vi "Measurement UI.vi"() -> ()   [LabVIEW 2021, in "Single Tone Measurements_Class D Amplifier.lvlib"]
uses:
  Single Tone Measurements_Class D Amplifier.lvlib
  shared/controls/units - snr.ctl
  shared/controls/units - ratio.ctl
  shared/controls/audio controls.lvlib
panel:
  in  "Graphs":enum32{"Frequency Domain", "Time Domain"}(tab)
  out "frequency domain":T1(graph)
  out "time domain":waveform(dbl)(graph)
  out "meas table":string[][](table)
  out "amplitude (Vrms)":dbl
  out "output power (W)":dbl
  in  "Configuration tab":enum32{"Protocol", "Measurement", "Units"}(tab)
  in  "master clock channel list":string caption="Master Clock Channel"
  in  "digital channel list":string caption="Digital Audio Channel"
  in  "logic level":enum32{"3.3 V", "1.8 V", "1.2 V"}(ring) caption="Logic level"
  in  "master clock rate":dbl=12288000.0 caption="Master clock rate" format="%#_6pHz"
  out "Bit clock rate":dbl=3072000.0 format="%#_6pHz"
  in  "number of channels":u8=2 caption="Number of channels"
  in  "TDM":bool
  in  "RJ":bool
  in  "LJ":bool
  in  "I2S":bool
  in  "bit clock edge sync":enum32{"Rising", "Falling"}(ring)=enum."Falling" caption="Bit clock edge sync"
  in  "frame clock rate":dbl=48000.0 caption="Frame clock rate" format="%#_6pHz"
  in  "data justification":enum32{"Left Justified", "Right Justified"}(ring) caption="Data justification"
  in  "endianness":enum32{"MSB First", "LSB First"}(ring) caption="Endianness"
  in  "bit depth":u8=24 caption="Bit depth"
  in  "channel length":u16=32 caption="Channel length"
  in  "frame sync edge for channel 0":enum32{"Rising", "Falling"}(ring)=enum."Falling" caption="Frame sync edge for Channel 0"
  in  "min settling cycles":u32 caption="Minimum settling cycles"
  in  "min settling time (s)":dbl=0.1 caption="Minimum settling time" format="%#_6ps"
  in  "min measurement cycles":u32 caption="Minimum measurement cycles"
  in  "min measurement time (s)":dbl=0.1 caption="Minimum measurement time" format="%#_6ps"
  in  "output power (W)":dbl=1.0 caption="Output power" format="%#_6p W"
  in  "output mode":enum16{"Level", "Power"}(ring) caption="Output mode"
  in  "Acquisition channel":tag
  in  "acq sampling rate":dbl=51200.0 caption="Sample rate" format="%#.6pHz"
  in  "lowpass filter":T2(ring) caption="Lowpass filter"
  in  "highpass filter":enum32{"DC", "AC"}(ring) caption="Highpass filter"
  in  "band start":dbl=20.0 caption="Band start" format="%#_6pHz"
  in  "band stop":dbl=20000.0 caption="Band stop" format="%#_6pHz"
  in  "weighting filter":T3(ring)=enum."A-weighting" caption="Weighting filter"
  in  "load impedance":dbl=4.0 caption="Load impedance" format="%#_6p Ohms"
  in  "output range (pk-pk)":dbl=15.0 caption="Output range" format="%.3p Vpk-pk"
  in  "signal frequency":dbl=1000.0 caption="Frequency" format="%#_6pHz"
  in  "output level (dB)":dbl=-1.0 caption="Output level" format="%#_6p dBFS"
  in  "testDBL":dbl
  in  "gain units":T4 caption="Gain"
  in  "THD units":T4 caption="THD"
  in  "THD+N units":T4 caption="THD+N"
  in  "SNR units":T5 caption="SNR"
  in  "channel 0 offset":u32=1
  out "fft - data":dbl[](array[numeric])
  out "fft - df":dbl
  out "fft - f0":dbl
  out "wfm - data":dbl[](array[numeric])
  out "wfm - dt":dbl
  out "wfm - t0":dbl
  out "SFDR (dBc)":dbl
  out "gain":dbl
  out "dynamic range (dB)":dbl
  out "THD":dbl
  out "THD+N":dbl
  out "SNR":dbl
  out "amplitude (dBFS)":dbl
  out "frequency (Hz)":dbl
  out "channel name":string
  in  "acq channel":string="PXI1Slot4/ai0"
  in  "signal phase":dbl caption="phase"
  # "hidden controls - used to sync with MeasLink"
  # "hidden indicators"
  # "Protocols"
  # "Audio Protocol"
  # "Clock Settings"
  # "Signal Level"
  # "Harware Resource"
  # "Filters"
  # "Output"
  # "Acquisition"
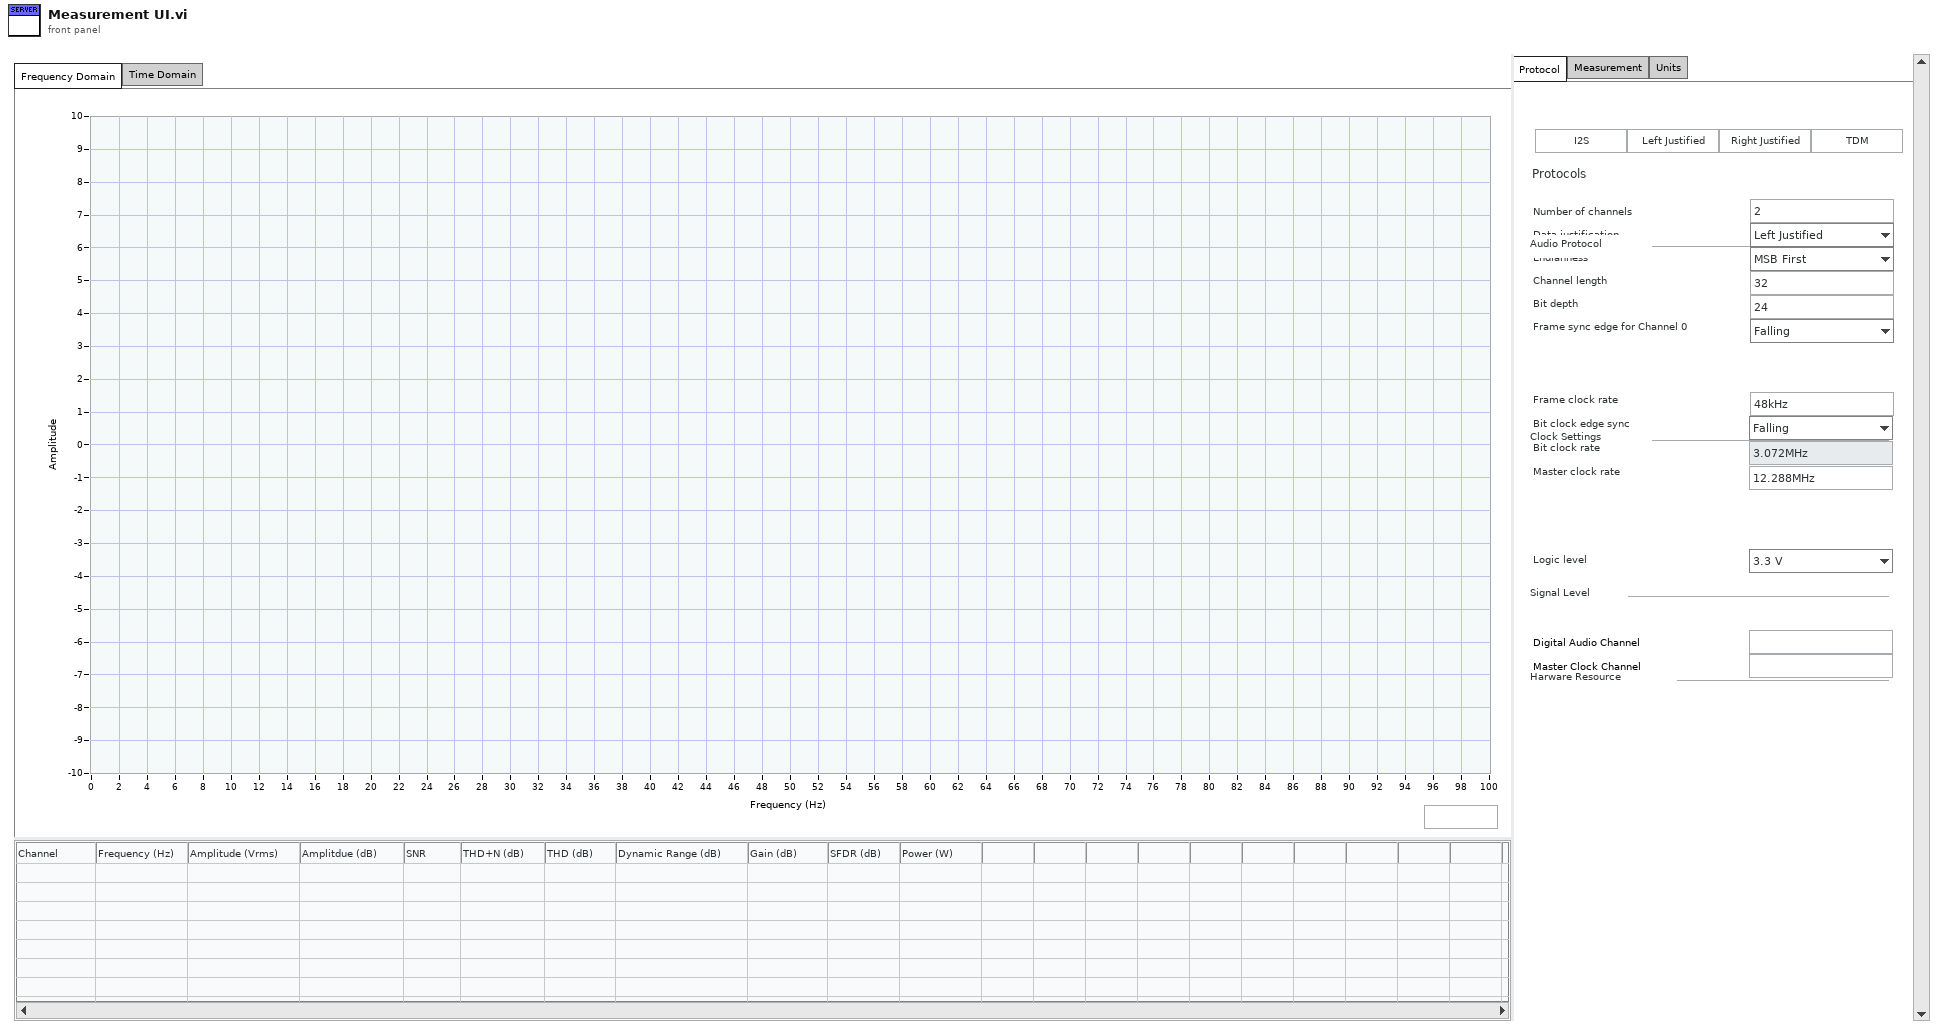
[diagram p1: front panel]
types:
  T1 = cluster{"fft - f0":dbl, "fft - df":dbl, "fft - data":dbl[]}
  T2 = enum32{"No filter", "AES17 20kHz", "AES17 40kHz"}
  T3 = enum32{"Linear", "A-weighting", "B-weighting", "C-weighting"}
  T4 = typedef "audio controls.lvlib/units - ratio.ctl" = enum16{"dB", "%", "x/y"}
  T5 = typedef "audio controls.lvlib/units - snr.ctl" = enum16{"dB", "x/y"}
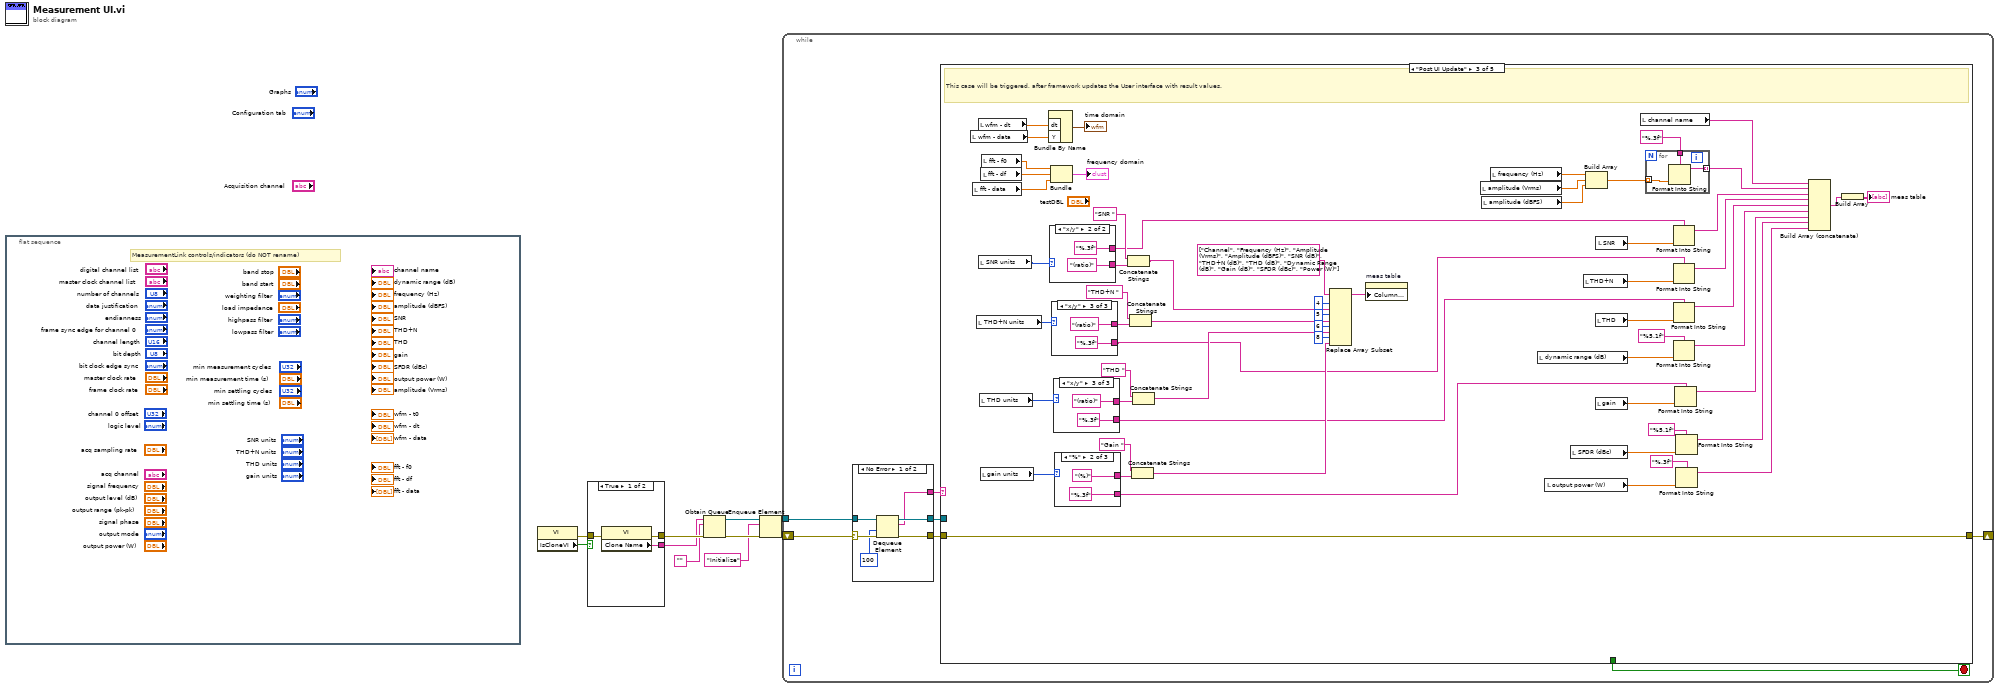
[diagram p0: block diagram]
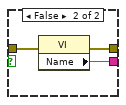
[diagram p2: hidden frame]
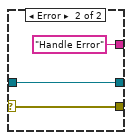
[diagram p3: hidden frame]
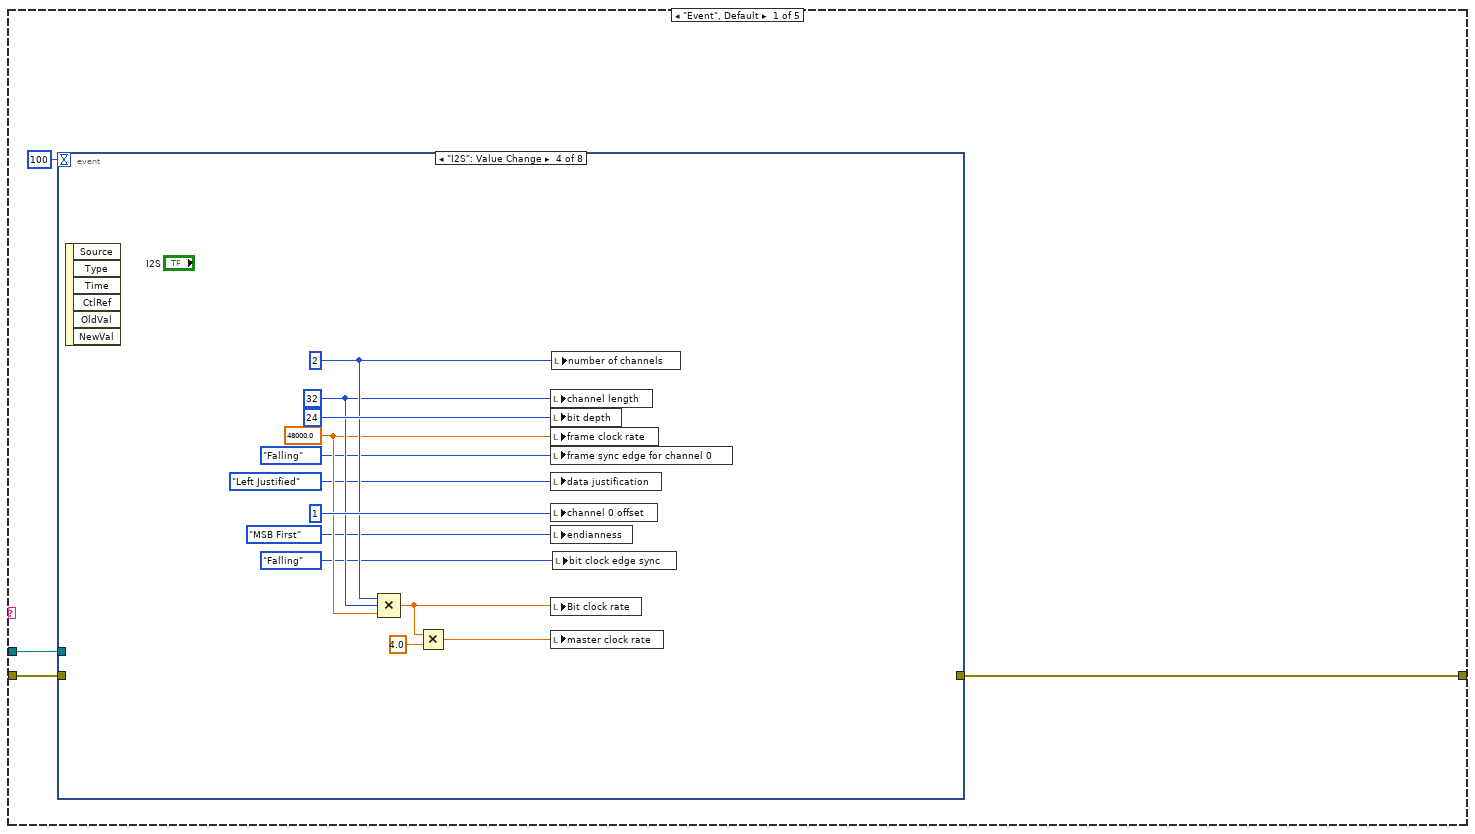
[diagram p4: hidden frame]
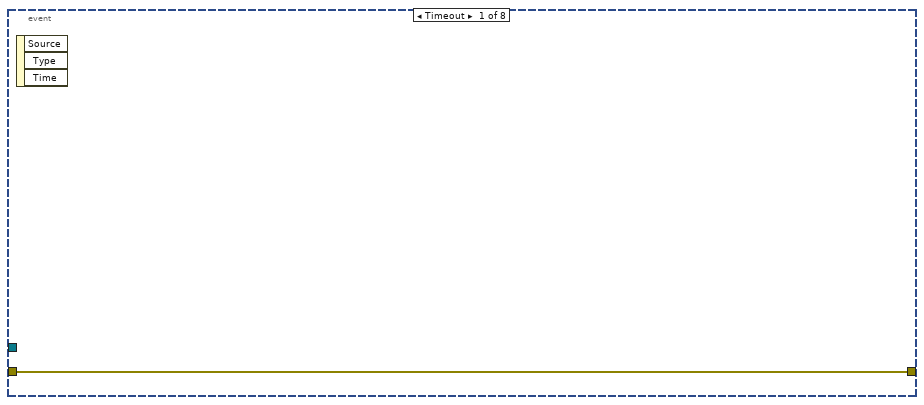
[diagram p5: hidden frame]
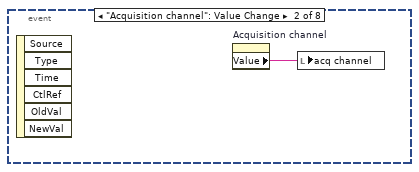
[diagram p6: hidden frame]
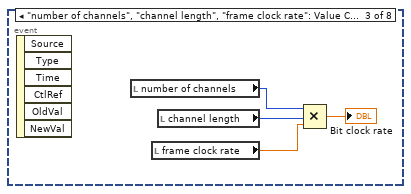
[diagram p7: hidden frame]
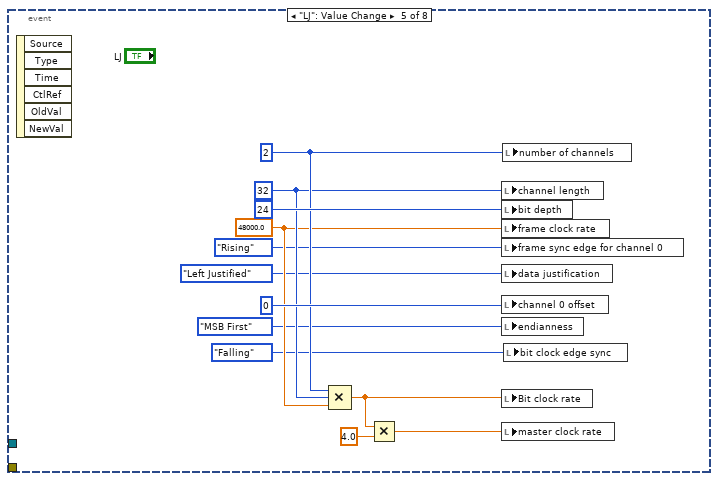
[diagram p8: hidden frame]
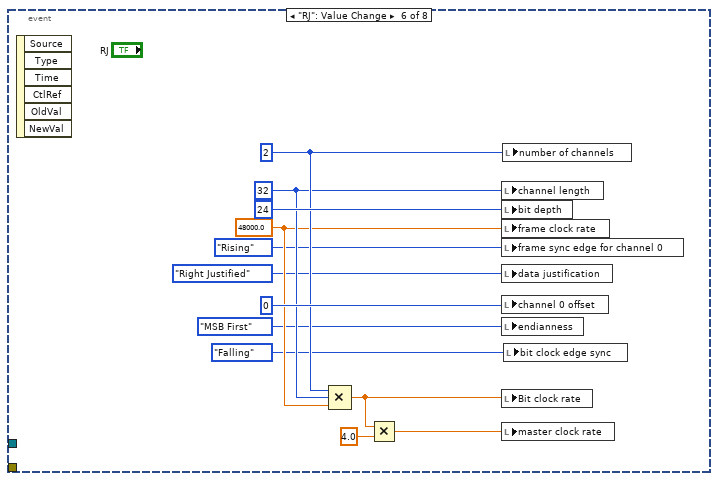
[diagram p9: hidden frame]
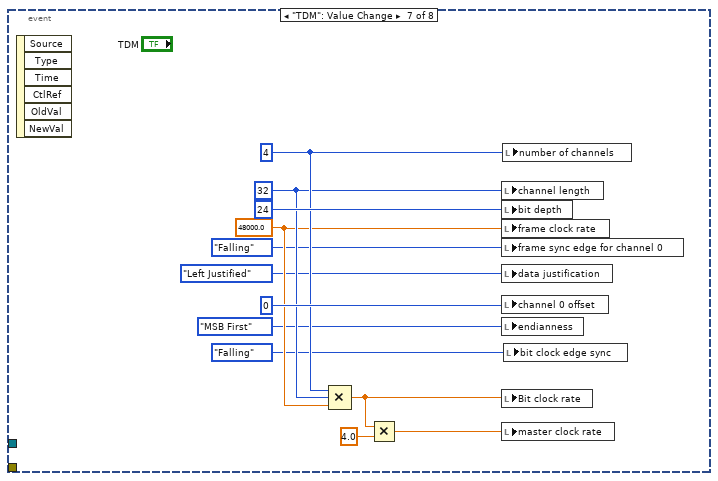
[diagram p10: hidden frame]
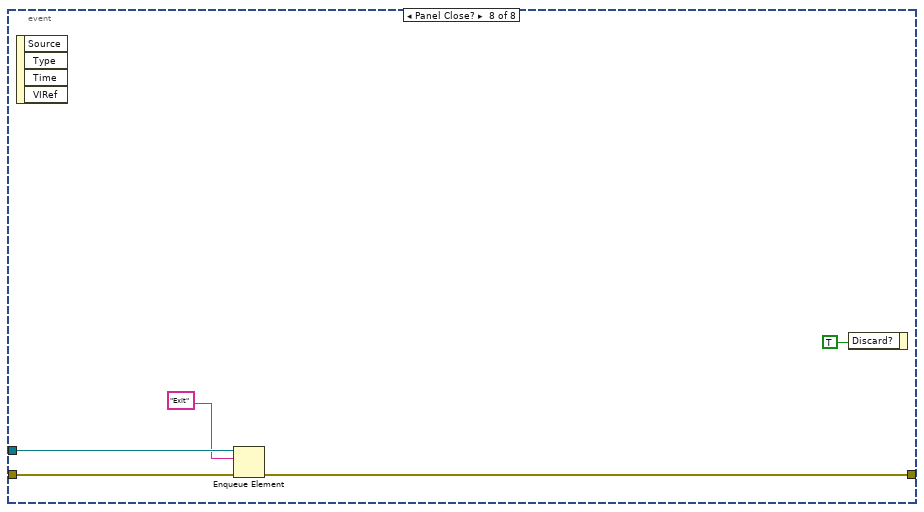
[diagram p11: hidden frame]
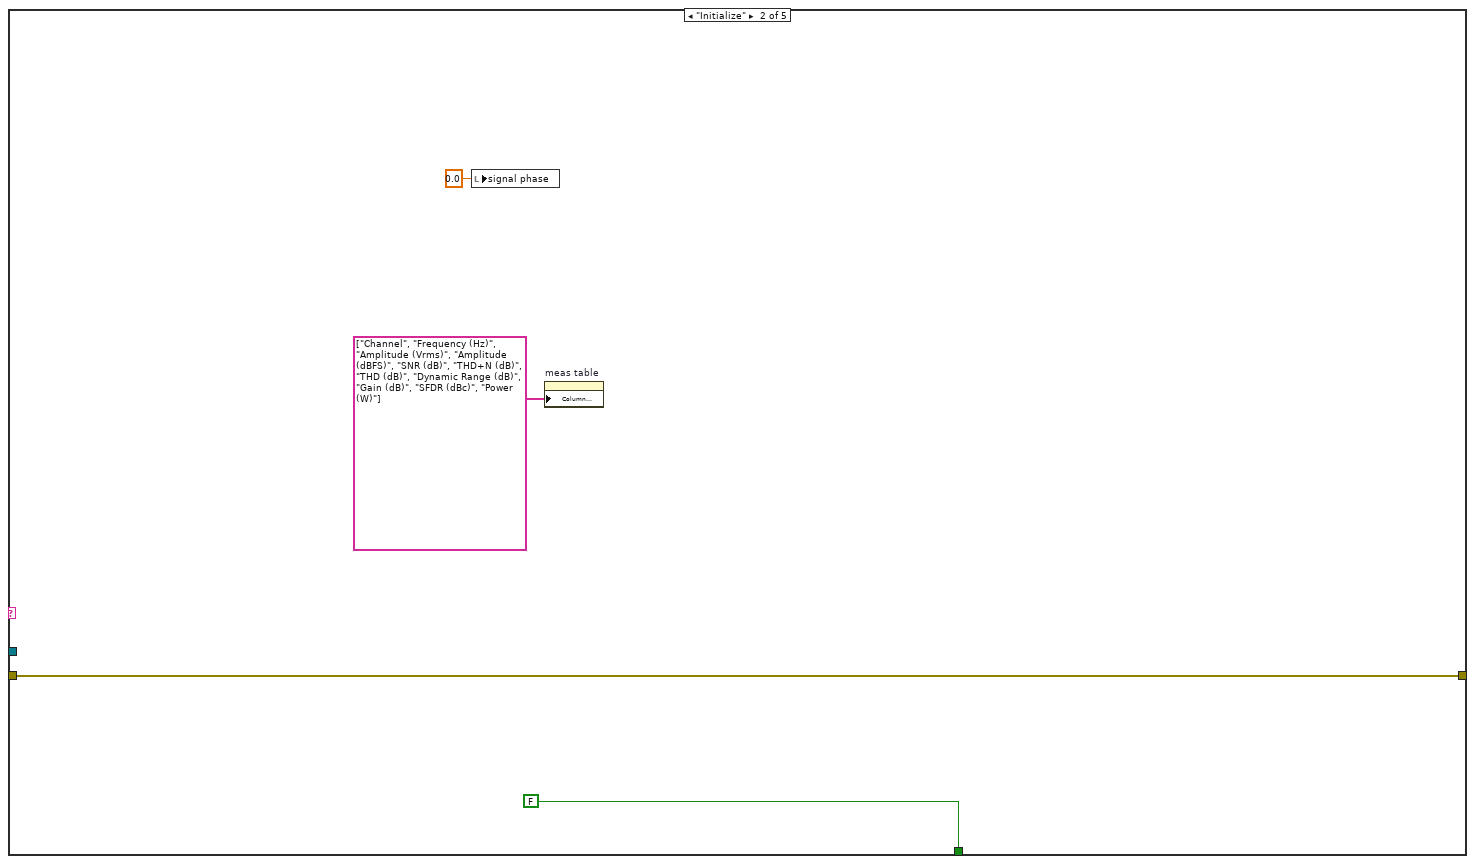
[diagram p12: hidden frame]
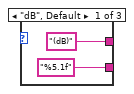
[diagram p13: hidden frame]
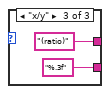
[diagram p14: hidden frame]
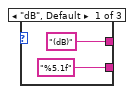
[diagram p15: hidden frame]
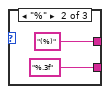
[diagram p16: hidden frame]
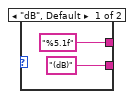
[diagram p17: hidden frame]
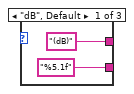
[diagram p18: hidden frame]
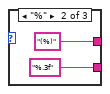
[diagram p19: hidden frame]
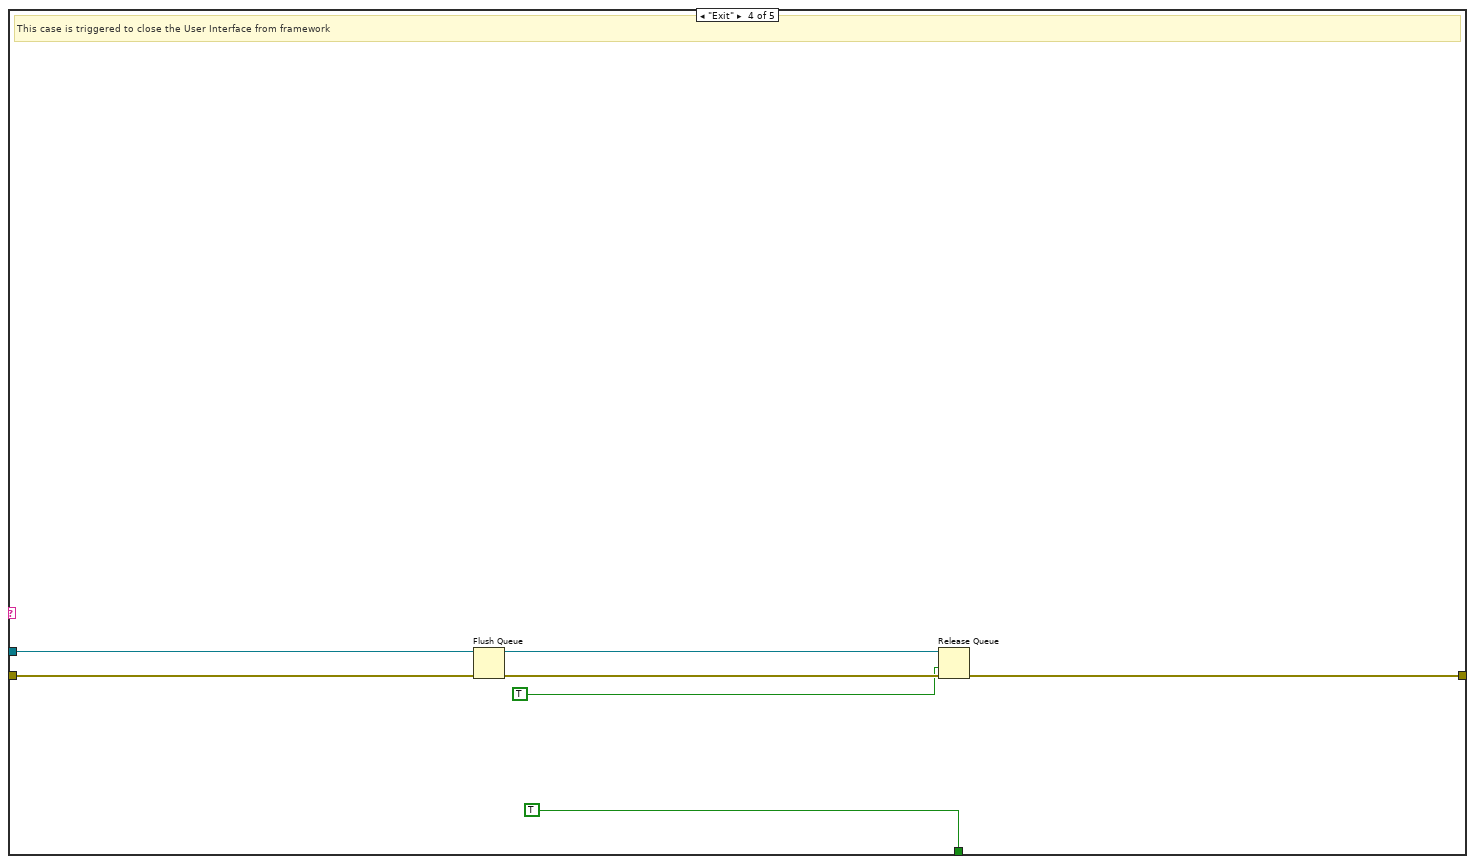
[diagram p20: hidden frame]
diagram:
  n1 = flat-sequence {
    frame #0 {
      # "MeasurementLink controls/indicators (do NOT rename)"
    }
  }
  n2 = property class="VI"() -> (error out=w1:errorcluster, "IsCloneVI"=w2:bool)  [unwired: 2 in, 1 out]
  n3 = case shown="True" w2 {
    tunnel: [w13 w16] -> w10
    tunnel: [w12 w15] -> w9
    tunnel: w1 -> [w11 w14]
    frame True {
      n4 = property class="VI"(error in=w11) -> (error out=w13:errorcluster, "Clone Name"=w12:string)  [unwired: 1 in, 1 out]
    }
    frame False {
      n5 = property class="VI"(error in=w14) -> (error out=w16:errorcluster, "Name"=w15:string)  [unwired: 1 in, 1 out]
    }
  }
  n6 = Obtain Queue(name (unnamed)=w9, element data type="", error in (no error)=w10) -> (queue out=w6:refnum<queue>, error out=w8:errorcluster)  [unwired: 2 in, 1 out]
  n7 = Enqueue Element(queue=w6, element="Initialize", error in (no error)=w8) -> (queue out=w5:refnum<queue>, error out=w7:errorcluster)  [unwired: 1 in, 1 out]
  n8 = while {
    shift-right: [w18] -> _
    shift-left: w7 -> [w23]
    tunnel: w5 -> [w21]
    stop <- w17 stop-if-true
    n9 = case shown="No Error" w23 {
      selector: w23 -> [w29 w32]
      tunnel: [w28 w32] -> w22
      tunnel: w21 -> [w27 w31]
      tunnel: [w26 w31] -> w20
      tunnel: [w25 "Handle Error"] -> w19
      frame No Error {
        n10 = Dequeue Element(queue=w27, timeout in ms (-1)=100, error in (no error)=w29) -> (queue out=w26:refnum<queue>, element=w25:string, error out=w28:errorcluster)  [unwired: 1 out]
      }
      frame Error {
      }
    }
    n11 = case shown="\"Post UI Update\"" w19 {
      tunnel: w22 -> [w35 w99 w159 w191 w192]
      tunnel: w20 -> [w33 _ _ w189 _]
      tunnel: [w36 w99 w159 w186 w192] -> w18
      tunnel: [_ FALSE _ TRUE _] -> w17
      frame "Event", Default {
        n12 = event shown="[3] \"I2S\": Value Change" {
          selector: _ -> [_ _ _ _ _ _ _ _]
          dyn-events: _ -> [_ _ _ _ _ _ _ _]
          timeout: 100 -> [_ _ _ _ _ _ _ _]
          tunnel: [w37 _ _ _ _ _ _ w93] -> w36
          tunnel: w35 -> [w37 _ _ _ _ _ _ w94]
          tunnel: w33 -> [_ _ _ _ _ _ _ w92]
          event Timeout {
            n13 = event-data() -> ()  [unwired: 1 in, 3 out]
          }
          event "Acquisition channel": Value Change {
            n14 = event-data() -> ()  [unwired: 1 in, 6 out]
            n15 = property on="Acquisition channel" class="DAQmxName"() -> ("Value"=w38:string)  [unwired: 2 in, 2 out]
            n16 = local write "acq channel"(w38) -> ()
          }
          event "number of channels", "channel length", "frame clock rate": Value Change {
            n17 = event-data() -> ()  [unwired: 1 in, 6 out]
            n18 = local read "number of channels"() -> (w42:u8)
            n19 = local read "frame clock rate"() -> (w40:dbl)
            n20 = local read "channel length"() -> (w41:u16)
            n21 = Compound Arithmetic op=MULTIPLY(w42, w41, w40) -> (→"Bit clock rate":dbl)
          }
          event "I2S": Value Change {
            w50 = 48000.0 ("Frame Clock Rate")
            w51 = u32 32 ("Channel Length")
            w52 = u32 2 ("Number of Channels")
            n22 = event-data() -> ()  [unwired: 1 in, 6 out]
            n23 = Compound Arithmetic op=MULTIPLY(w52, w51, w50) -> (w49:dbl)
            n24 = Multiply(x=w49, y=4.0) -> (x*y=w48:dbl)
            n25 = local write "channel length"(w51) -> ()
            n26 = local write "bit depth"(u32 24 ("Bit Depth")) -> ()
            n27 = local write "frame clock rate"(w50) -> ()
            n28 = local write "frame sync edge for channel 0"(enum32{"Rising", "Falling"}."Falling" ("bit clock edge sync")) -> ()
            n29 = local write "data justification"(enum32{"Left Justified", "Right Justified"}."Left Justified" ("data justification")) -> ()
            n30 = local write "channel 0 offset"(u32 1 ("Channel 0 Offset")) -> ()
            n31 = local write "endianness"(enum32{"MSB First", "LSB First"}."MSB First" ("endianness")) -> ()
            n32 = local write "Bit clock rate"(w49) -> ()
            n33 = local write "master clock rate"(w48) -> ()
            n34 = local write "number of channels"(w52) -> ()
            n35 = local write "bit clock edge sync"(enum32{"Rising", "Falling"}."Falling" ("frame sync edge for channel 0")) -> ()
          }
          event "LJ": Value Change {
            w62 = 48000.0 ("Frame Clock Rate")
            w63 = u32 32 ("Channel Length")
            w64 = u32 2 ("Number of Channels")
            n36 = event-data() -> ()  [unwired: 1 in, 6 out]
            n37 = Compound Arithmetic op=MULTIPLY(w64, w63, w62) -> (w61:dbl)
            n38 = Multiply(x=w61, y=4.0) -> (x*y=w60:dbl)
            n39 = local write "channel length"(w63) -> ()
            n40 = local write "bit depth"(u32 24 ("Bit Depth")) -> ()
            n41 = local write "frame clock rate"(w62) -> ()
            n42 = local write "frame sync edge for channel 0"(enum32{"Rising", "Falling"}."Rising" ("bit clock edge sync")) -> ()
            n43 = local write "data justification"(enum32{"Left Justified", "Right Justified"}."Left Justified" ("data justification")) -> ()
            n44 = local write "channel 0 offset"(u32 0 ("Channel 0 Offset")) -> ()
            n45 = local write "endianness"(enum32{"MSB First", "LSB First"}."MSB First" ("endianness")) -> ()
            n46 = local write "Bit clock rate"(w61) -> ()
            n47 = local write "master clock rate"(w60) -> ()
            n48 = local write "number of channels"(w64) -> ()
            n49 = local write "bit clock edge sync"(enum32{"Rising", "Falling"}."Falling" ("frame sync edge for channel 0")) -> ()
          }
          event "RJ": Value Change {
            w74 = 48000.0 ("Frame Clock Rate")
            w75 = u32 32 ("Channel Length")
            w76 = u32 2 ("Number of Channels")
            n50 = event-data() -> ()  [unwired: 1 in, 6 out]
            n51 = Compound Arithmetic op=MULTIPLY(w76, w75, w74) -> (w73:dbl)
            n52 = Multiply(x=w73, y=4.0) -> (x*y=w72:dbl)
            n53 = local write "channel length"(w75) -> ()
            n54 = local write "bit depth"(u32 24 ("Bit Depth")) -> ()
            n55 = local write "frame clock rate"(w74) -> ()
            n56 = local write "frame sync edge for channel 0"(enum32{"Rising", "Falling"}."Rising" ("bit clock edge sync")) -> ()
            n57 = local write "data justification"(enum32{"Left Justified", "Right Justified"}."Right Justified" ("data justification")) -> ()
            n58 = local write "channel 0 offset"(u32 0 ("Channel 0 Offset")) -> ()
            n59 = local write "endianness"(enum32{"MSB First", "LSB First"}."MSB First" ("endianness")) -> ()
            n60 = local write "Bit clock rate"(w73) -> ()
            n61 = local write "master clock rate"(w72) -> ()
            n62 = local write "number of channels"(w76) -> ()
            n63 = local write "bit clock edge sync"(enum32{"Rising", "Falling"}."Falling" ("frame sync edge for channel 0")) -> ()
          }
          event "TDM": Value Change {
            w86 = 48000.0 ("Frame Clock Rate")
            w87 = u32 32 ("Channel Length")
            w88 = u32 4 ("Number of Channels")
            n64 = event-data() -> ()  [unwired: 1 in, 6 out]
            n65 = Compound Arithmetic op=MULTIPLY(w88, w87, w86) -> (w85:dbl)
            n66 = Multiply(x=w85, y=4.0) -> (x*y=w84:dbl)
            n67 = local write "channel length"(w87) -> ()
            n68 = local write "bit depth"(u32 24 ("Bit Depth")) -> ()
            n69 = local write "frame clock rate"(w86) -> ()
            n70 = local write "frame sync edge for channel 0"(enum32{"Rising", "Falling"}."Falling" ("bit clock edge sync")) -> ()
            n71 = local write "data justification"(enum32{"Left Justified", "Right Justified"}."Left Justified" ("data justification")) -> ()
            n72 = local write "channel 0 offset"(u32 0 ("Channel 0 Offset")) -> ()
            n73 = local write "endianness"(enum32{"MSB First", "LSB First"}."MSB First" ("endianness")) -> ()
            n74 = local write "Bit clock rate"(w85) -> ()
            n75 = local write "master clock rate"(w84) -> ()
            n76 = local write "number of channels"(w88) -> ()
            n77 = local write "bit clock edge sync"(enum32{"Rising", "Falling"}."Falling" ("frame sync edge for channel 0")) -> ()
          }
          event Panel Close? {
            n78 = event-data() -> ()  [unwired: 1 in, 4 out]
            n79 = Enqueue Element(queue=w92, element="Exit", error in (no error)=w94) -> (error out=w93:errorcluster)  [unwired: 1 in, 2 out]
            n80 = event-data("Discard?"=TRUE) -> ()  [unwired: 1 in, 1 out]
          }
        }
      }
      frame "Initialize" {
        n81 = local write "signal phase"(0.0 ("signal phase")) -> ()
        n82 = property on="meas table" class="Tbl (strict)"("Column Headers[]"=string[] ["Channel", "Frequency (Hz)", "Amplitude (Vrms)", "Amplitude (dBFS)", "SNR (dB)", "THD+N (dB)", "THD (dB)", "Dynamic Range (dB)", "Gain (dB)", "SFDR (dBc)", "Power (W)"] ("Column Header Strings[]")) -> ()  [unwired: 2 in, 2 out]
      }
      frame "Post UI Update" {
        # "This case will be triggered, after framework updates the User interface with result values."
        n83 = local read "wfm - data"() -> (w157:dbl[])
        n84 = local read "fft - data"() -> (w153:dbl[])
        n85 = local read "THD+N units"() -> (w132:T4)
        n86 = local read "wfm - dt"() -> (w158:dbl)
        n87 = local read "SNR units"() -> (w115:T5)
        n88 = local read "THD units"() -> (w105:T4)
        n89 = local read "gain units"() -> (w103:T4)
        n90 = local read "fft - df"() -> (w154:dbl)
        n91 = local read "fft - f0"() -> (w155:dbl)
        n92 = Bundle By Name("dt"=w158, "Y"=w157) -> (→"time domain":waveform(dbl))  [unwired: 1 in]
        n93 = case shown="\"x/y\"" w115 {
          tunnel: ["(dB)" "(ratio)"] -> w131
          tunnel: ["%5.1f" ("initial string") "%.3f" ("initial string")] -> w114
          frame "dB", Default {
          }
          frame "x/y" {
          }
        }
        n94 = Bundle("fft - f0"=w155, "fft - df"=w154, "fft - data"=w153) -> (→"frequency domain":T1)  [unwired: 1 in]
        n95 = case shown="\"x/y\"" w132 {
          tunnel: ["(dB)" "(%)" "(ratio)"] -> w134
          tunnel: ["%5.1f" ("initial string") "%.3f" ("initial string") "%.3f" ("initial string")] -> w102
          frame "dB", Default {
          }
          frame "%" {
          }
          frame "x/y" {
          }
        }
        n96 = case shown="\"x/y\"" w105 {
          tunnel: ["(dB)" "(%)" "(ratio)"] -> w106
          tunnel: ["%5.1f" ("initial string") "%.3f" ("initial string") "%.3f" ("initial string")] -> w101
          frame "dB", Default {
          }
          frame "%" {
          }
          frame "x/y" {
          }
        }
        n97 = case shown="\"%\"" w103 {
          tunnel: ["(dB)" "(%)" "(ratio)"] -> w104
          tunnel: ["%5.1f" ("initial string") "%.3f" ("initial string") "%.3f" ("initial string")] -> w100
          frame "dB", Default {
          }
          frame "%" {
          }
          frame "x/y" {
          }
        }
        n98 = Concatenate Strings("SNR " ("string"), w131) -> (w127:string)
        n99 = Concatenate Strings("THD+N " ("string"), w134) -> (w126:string)
        n100 = Concatenate Strings("Gain " ("string"), w104) -> (w124:string)
        n101 = Concatenate Strings("THD " ("string"), w106) -> (w125:string)
        n102 = Replace Array Subset(array=string[] ["Channel", "Frequency (Hz)", "Amplitude (Vrms)", "Amplitude (dBFS)", "SNR (dB)", "THD+N (dB)", "THD (dB)", "Dynamic Range (dB)", "Gain (dB)", "SFDR (dBc)", "Power (W)"] ("Column Header Strings[]"), new element #1=w127, index #1=4 ("index"), new element #2=w126, index #2=5 ("index"), new element #3=w125, index #3=6 ("index"), new element #4=w124, index #4=8 ("index")) -> (w128:string[])
        n103 = property on="meas table" class="Tbl (strict)"("Column Headers[]"=w128) -> ()  [unwired: 2 in, 2 out]
        n104 = local read "amplitude (Vrms)"() -> (w118:dbl)
        n105 = local read "amplitude (dBFS)"() -> (w119:dbl)
        n106 = local read "frequency (Hz)"() -> (w143:dbl)
        n107 = local read "dynamic range (dB)"() -> (w111:dbl)
        n108 = local read "output power (W)"() -> (w139:dbl)
        n109 = local read "SFDR (dBc)"() -> (w141:dbl)
        n110 = local read "THD+N"() -> (w113:dbl)
        n111 = Build Array(w143, w118, w119) -> (w150:dbl[])
        n112 = local read "THD"() -> (w112:dbl)
        n113 = local read "gain"() -> (w142:dbl)
        n114 = local read "SNR"() -> (w116:dbl)
        n115 = local read "channel name"() -> (w140:string)
        n116 = for {
          tunnel: w150 -> [w182] mode=indexing
          tunnel: "%.3f" ("initial string") -> [w183]
          tunnel: [w184] -> w149 mode=indexing
          n117 = Format Into String(format string=w183, w182) -> (resulting string=w184:string)  [unwired: 2 in, 1 out]
        }
        n118 = Format Into String(format string=w114, w116) -> (resulting string=w117:string)  [unwired: 2 in, 1 out]
        n119 = Format Into String(format string=w102, w113) -> (resulting string=w107:string)  [unwired: 2 in, 1 out]
        n120 = Format Into String(format string=w101, w112) -> (resulting string=w108:string)  [unwired: 2 in, 1 out]
        n121 = Format Into String(format string="%5.1f" ("initial string"), w111) -> (resulting string=w109:string)  [unwired: 2 in, 1 out]
        n122 = Format Into String(format string=w100, w142) -> (resulting string=w147:string)  [unwired: 2 in, 1 out]
        n123 = Format Into String(format string="%5.1f" ("initial string"), w141) -> (resulting string=w146:string)  [unwired: 2 in, 1 out]
        n124 = Format Into String(format string="%.3f" ("initial string"), w139) -> (resulting string=w137:string)  [unwired: 2 in, 1 out]
        n125 = Build Array (concatenate)(w140, w149, w117, w107, w108, w109, w147, w146, w137) -> (w148:string[])
        n126 = Build Array(w148) -> (→"meas table":string[][])
      }
      frame "Exit" {
        # "This case is triggered to close the User Interface from framework"
        n127 = Flush Queue(queue=w189, error in (no error)=w191) -> (queue out=w188:refnum<queue>, error out=w187:errorcluster)  [unwired: 1 out]
        n128 = Release Queue(queue=w188, force destroy? (F)=TRUE, error in (no error)=w187) -> (error out=w186:errorcluster)  [unwired: 2 out]
      }
      frame "Handle Error" {
      }
    }
  }
